vi "Config Type.vi"(11 "Event Command in":refnum<class "Event Command.lvclass">) -> (2 "Command Config Type":refnum<class "Command Config.lvclass">)   [LabVIEW 2020, in "VolatusSeq.lvlib" / "Event Command.lvclass"]
uses:
  Event Command.lvclass
  Event Command.lvclass/Event Command.ctl
  VolatusSeqConfig/Event Command Config/Event Command Config.lvclass
  C:/dev/lv20CE/relink/lv-volatus/VolatusSeqConfig/Command Config/Command Config.lvclass
  C:/dev/lv20CE/relink/lv-volatus/VolatusSeqConfig/Event Command Config/Event Command Config.lvclass
  VolatusSeqConfig/Command Config/Command Config.lvclass
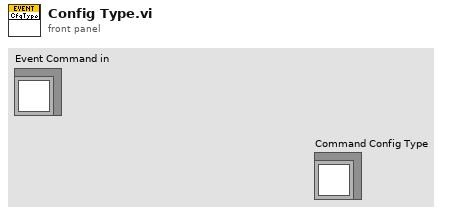
[diagram p1: front panel]
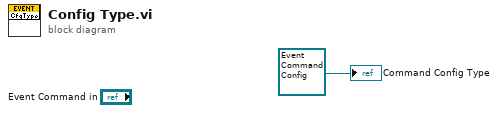
[diagram p0: block diagram]
diagram:
  "Command Config Type" <- refnum<class "Event Command Config.lvclass"> refnum ("VolatusSeqConfig.lvlib:Event Command Config.lvclass")
